vi "MoAgSy_Message.appendData2Variant.vi"(0 "initData":variant, 1 "addressee":string, 2 "type":enum16{"mobile Agent", "Visitor", "Message"}(ring)=enum."Message", 3 "Object":refnum<class>, 4 "request reply":bool, 5 "error in":errorcluster, 6 "gpg crypted":bool, 7 "sender":string, 8 "message":string, 9 "reply to":string, 11 "reply id":string) -> (14 "dup_initData":variant, 19 "error out":errorcluster)   [LabVIEW 2009, in "MoAgSy.lvlib" / "MoAgSy_Message.lvclass"]
uses:
  MoAgSy_Message.lvclass
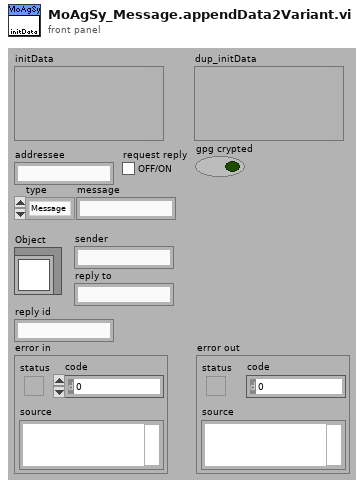
[diagram p1: front panel]
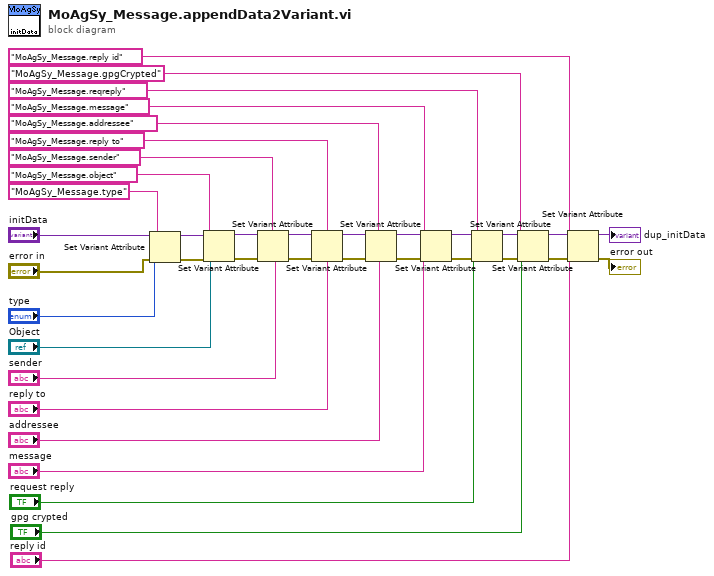
[diagram p0: block diagram]
diagram:
  n1 = Set Variant Attribute(Variant="initData", name="MoAgSy_Message.type", value="type", error in="error in") -> (Variant out=w34:variant, error out=w35:errorcluster)  [unwired: 1 out]
  n2 = Set Variant Attribute(Variant=w34, name="MoAgSy_Message.object", value="Object", error in=w35) -> (Variant out=w30:variant, error out=w31:errorcluster)  [unwired: 1 out]
  n3 = Set Variant Attribute(Variant=w30, name="MoAgSy_Message.sender", value="sender", error in=w31) -> (Variant out=w26:variant, error out=w27:errorcluster)  [unwired: 1 out]
  n4 = Set Variant Attribute(Variant=w26, name="MoAgSy_Message.reply to", value="reply to", error in=w27) -> (Variant out=w22:variant, error out=w23:errorcluster)  [unwired: 1 out]
  n5 = Set Variant Attribute(Variant=w22, name="MoAgSy_Message.addressee", value="addressee", error in=w23) -> (Variant out=w17:variant, error out=w18:errorcluster)  [unwired: 1 out]
  n6 = Set Variant Attribute(Variant=w17, name="MoAgSy_Message.message", value="message", error in=w18) -> (Variant out=w14:variant, error out=w13:errorcluster)  [unwired: 1 out]
  n7 = Set Variant Attribute(Variant=w14, name="MoAgSy_Message.reqreply", value="request reply", error in=w13) -> (Variant out=w10:variant, error out=w9:errorcluster)  [unwired: 1 out]
  n8 = Set Variant Attribute(Variant=w10, name="MoAgSy_Message.gpgCrypted", value="gpg crypted", error in=w9) -> (Variant out=w6:variant, error out=w4:errorcluster)  [unwired: 1 out]
  n9 = Set Variant Attribute(Variant=w6, name="MoAgSy_Message.reply id", value="reply id", error in=w4) -> (Variant out=→"dup_initData":variant, error out=→"error out":errorcluster)  [unwired: 1 out]
